vi "XML Script - Append Terminal Name (GrowableFunction).vi"(4 "i-th term":i32, 5 "name":string) -> (2 "name.element[i]":string)   [LabVIEW 2020]
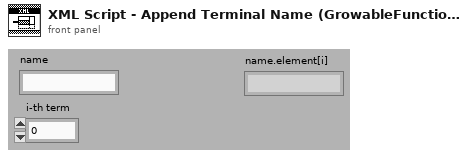
[diagram p1: front panel]
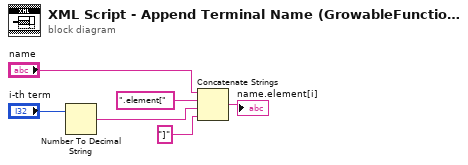
[diagram p0: block diagram]
diagram:
  n1 = Number To Decimal String(number="i-th term") -> (decimal integer string=w3:string)  [unwired: 1 in]
  n2 = Concatenate Strings("name", ".element[" ("string"), w3, "]" ("string")) -> (→"name.element[i]":string)
